vi "SearchUSB.vi"(8 "error in":errorcluster, 10 "USB":string) -> (0 "error out":errorcluster, 2 "USBPort":refnum<visa-resource-name>)   [LabVIEW 2013]
uses:
  <vilib>/registry/registry.llb/Registry SAM.ctl
  <vilib>/registry/registry.llb/Registry RtKey.ctl
  <vilib>/registry/registry.llb/Read Registry Value Simple STR.vi
panel:
  out "为空？":bool
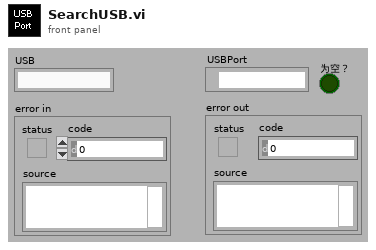
[diagram p1: front panel]
types:
  T1 = typedef "Registry RtKey.ctl" = enum32{"HKEY_CLASSES_ROOT", "HKEY_CURRENT_USER", "HKEY_LOCAL_MACHINE", "HKEY_USERS", "HKEY_PERFORMANCE_DATA", "HKEY_CURRENT_CONFIG", "HKEY_DYN_DATA"}
  T2 = typedef "Registry SAM.ctl" = enum32{"KEY_QUERY_VALUE", "KEY_SET_VALUE", "KEY_CREATE_SUB_KEY", "KEY_ENUMERATE_SUB_KEYS", "KEY_NOTIFY", "KEY_CREATE_LINK", "KEY_READ", "KEY_WRITE", "KEY_ALL_ACCESS", "KEY_READ | KEY_WRITE"}
  T3 = typedef "Registry refnum.ctl" = refnum<k1>
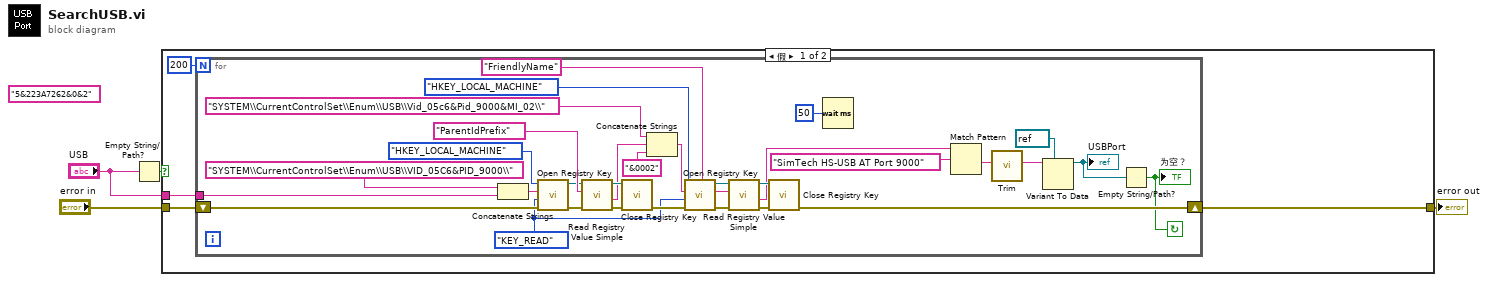
[diagram p0: block diagram]
diagram:
  (unwired) "5&223A7262&0&2" ("正则表达式")
  n1 = Empty String/Path?(string/path="USB") -> (empty?=w1:bool)
  n2 = case shown="假" w1 {
    tunnel: "error in" -> [w8 w40]
    tunnel: [w6 w40] -> w4
    tunnel: "USB" -> [w7 _]
    frame False {
      n3 = for {
        N: 200 -> [_]
        tunnel: w7 -> [w33]
        shift-right: [w21] -> w6
        shift-left: w8 -> [w36]
        stop <- w10 continue-if-true
        w15 = Registry_SAM."KEY_READ" ("security access mask (KEY_READ | KEY_WRITE)")
        n4 = Concatenate Strings("SYSTEM\\CurrentControlSet\\Enum\\USB\\VID_05C6&PID_9000\\" ("subkey"), w33) -> (w38:string)
        n5 = call <vilib>:"Open Registry Key.vi"("error in (no error)"=w36, "security access mask (KEY_READ | KEY_WRITE)"=w15, "subkey"=w38, "root key (HKEY_LOCAL_MACHINE)"=Registry_RtKey."HKEY_LOCAL_MACHINE") -> ("error out"=w32:errorcluster, "refnum out"=w31:T3)  [unwired: 6 out]
        n6 = call-poly <vilib>:"Read Registry Value Simple.vi"("error in (no error)"=w32, "value"="ParentIdPrefix", "refnum"=w31) -> ("error out"=w35:errorcluster, "String/Binary data"=w19:string, "refnum out"=w30:T3)  [unwired: 1 in, 3 out]
        n7 = call <vilib>:"Close Registry Key.vi"("error in (no error)"=w35, "refnum"=w30) -> ("error out"=w22:errorcluster)  [unwired: 5 out]
        n8 = Concatenate Strings("SYSTEM\\CurrentControlSet\\Enum\\USB\\Vid_05c6&Pid_9000&MI_02\\" ("subkey"), w19, "&0002" ("字符串")) -> (w23:string)
        n9 = call <vilib>:"Open Registry Key.vi"("error in (no error)"=w22, "security access mask (KEY_READ | KEY_WRITE)"=w15, "subkey"=w23, "root key (HKEY_LOCAL_MACHINE)"=Registry_RtKey."HKEY_LOCAL_MACHINE") -> ("error out"=w27:errorcluster, "refnum out"=w28:T3)  [unwired: 6 out]
        n10 = call-poly <vilib>:"Read Registry Value Simple.vi"("error in (no error)"=w27, "value"="FriendlyName", "refnum"=w28) -> ("error out"=w25:errorcluster, "String/Binary data"=w18:string, "refnum out"=w29:T3)  [unwired: 1 in, 3 out]
        n11 = call <vilib>:"Close Registry Key.vi"("error in (no error)"=w25, "refnum"=w29) -> ("error out"=w21:errorcluster)  [unwired: 5 out]
        n12 = Wait (ms)(milliseconds to wait=u32 50 ("等待时间（毫秒）")) -> ()  [unwired: 1 out]
        n13 = Match Pattern(string=w18, regular expression="SimTech HS-USB AT Port 9000" ("正则表达式")) -> (after substring=w11:string)  [unwired: 4 out]
        n14 = call "Trim.vi"("String"=w11) -> ("TrimStr"=w13:string)  [unwired: 10 in]
        n15 = Variant To Data(type=refnum<visa-resource-name> refnum ("VISA resource name"), Variant=w13) -> (data=w12:refnum<visa-resource-name>)  [unwired: 1 in, 1 out]
        "USBPort" <- w12
        n16 = Empty String/Path?(string/path=w12) -> (empty?=w10:bool)
        "为空？" <- w10
      }
    }
    frame True {
    }
  }
  "error out" <- w4
